vi "test_MultipleSessionsReserved_CallCloseSessions_ConnectionMapSessionsCleared.vi"(8 "error in":errorcluster) -> (0 "error out":errorcluster, 2 "result":string, 3 "pass":bool)   [LabVIEW 2020, in "MeasurementServerTests.lvlib"]
uses:
  MeasurementServerTests.lvlib
  Runtime/MeasurementLink Session Management/Session Reservation/Connection with Session.ctl
  Runtime/MeasurementLink Session Management/Session Reservation/Connection.ctl
  816d9199-244a-4674-a692-355e6ad76c7e.vi
  3a73e73b-7889-4e8d-bfa9-c59269005a4e.vi
  Helpers/Fake Instrument/Fake Instrument.lvclass
  C:/dev/measurementlink-labview/Source/Runtime/MeasurementLink Instrument/IInstrument/IInstrument.lvclass
  Runtime/MeasurementLink Session Management/Session Reservation/Get Connections Dispatcher.vi
  Runtime/MeasurementLink Session Management/Session Reservation/Session Reservation.lvclass
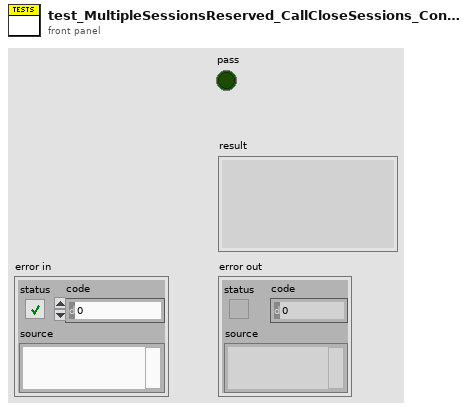
[diagram p1: front panel]
types:
  T1 = typedef "MeasurementLink Session Management.lvlib/Session Reservation.lvclass/Connection with Session.ctl" = cluster{"connection":T2, "session":variant}
  T2 = typedef "MeasurementLink Session Management.lvlib/Session Reservation.lvclass/Connection.ctl" = cluster{"pin or relay name":string, "site":i32, "instrument type id":string, "channel":string}
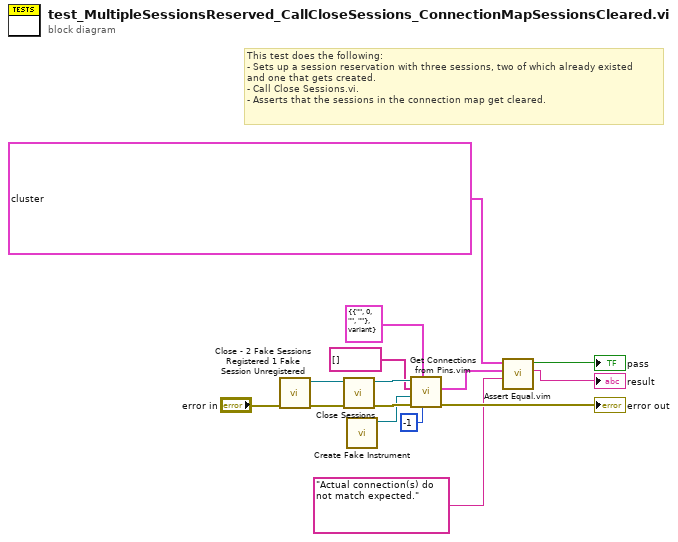
[diagram p0: block diagram]
diagram:
  # "This test does the following:\n- Sets up a session reservation with three sessions, two of which already existed\nand one that gets created.\n- Call Close Sessions.vi.\n- Asserts that the sessions in the connection map get cleared."
  n1 = call "Close - 2 Fake Sessions Registered 1 Fake Session Unregistered.vi"("error in (no error)"="error in") -> ("error out"=w14:errorcluster, "Session Reservation out"=w13:refnum<class "Session Reservation.lvclass">)  [unwired: 9 in]
  n2 = call "Close Sessions.vi"("error in"=w14, "session reservation in"=w13) -> ("error out"=w12:errorcluster, "session reservation out"=w11:refnum<class "Session Reservation.lvclass">)  [unwired: 8 in]
  n3 = call "Create Fake Instrument.vi"() -> ("fake instrument out"=w1:refnum<class "Fake Instrument.lvclass">)  [unwired: 10 in, 1 out]
  n4 = call "Get Connections from Pins.vim"("site"=-1, "connection type"=T1 {"connection"={"pin or relay name"="", "site"=0, "instrument type id"="", "channel"=""}, "session"=variant}, "error in"=w12, "instrument"=w1, "pin or relay names"=string[] [], "session reservation in"=w11) -> ("error out"=→"error out":errorcluster, "connections"=w6:T1[])  [unwired: 3 in, 1 out]
  n5 = call "Assert Equal.vim"("failure message"="Actual connection(s) do not match expected.", "actual value"=w6, "expected value"=T1[] [{"connection"={"pin or relay name"="PinA", "site"=4, "instrument type id"="fake_instrument_type", "channel"="1"}, "session"=variant}, {"connection"={"pin or relay name"="PinB", "site"=4, "instrument type id"="fake_instrument_type", "channel"="0"}, "session"=variant}, {"connection"={"pin or relay name"="PinC", "site"=4, "instrument type id"="fake_instrument_type", "channel"="2"}, "session"=variant}] ("connections")) -> ("message"=→"result":string, "equal?"=→"pass":bool)  [unwired: 7 in]
